vi "Aggregate to Test Suite.vi"(8 "error in (no error)":errorcluster, 11 "Test Finder In":refnum<class "Test Finder.lvclass">) -> (0 "error out":errorcluster, 2 "Test Suite":refnum<class "LUnit Test Suite.lvclass">, 3 "Test Finder Out":refnum<class "Test Finder.lvclass">)   [LabVIEW 2020, in "Test Finder.lvclass"]
uses:
  Test Finder.lvclass
  Test Suite/LUnit Test Suite.lvclass
  Test Finder.lvclass/Test Finder.ctl
  Test Case/LUnit Test Case.lvclass
  Test Case/LUnit Test Case.lvclass/LUnit Test Case.ctl
  Test Suite/LUnit Test Suite.lvclass/LUnit Test Suite.ctl
  Test Case/Public/Accessors/Read Enabled Test Methods.vi
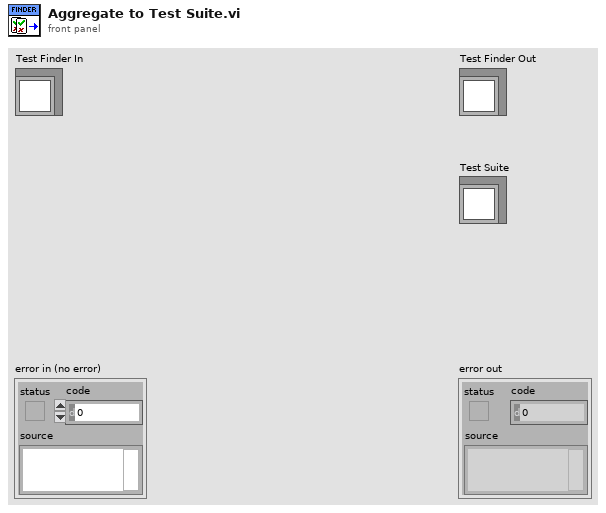
[diagram p1: front panel]
types:
  T1 = map{string, cluster{"Dynamic Methods":map{string, path}, "Static Methods":map{string, path}}}
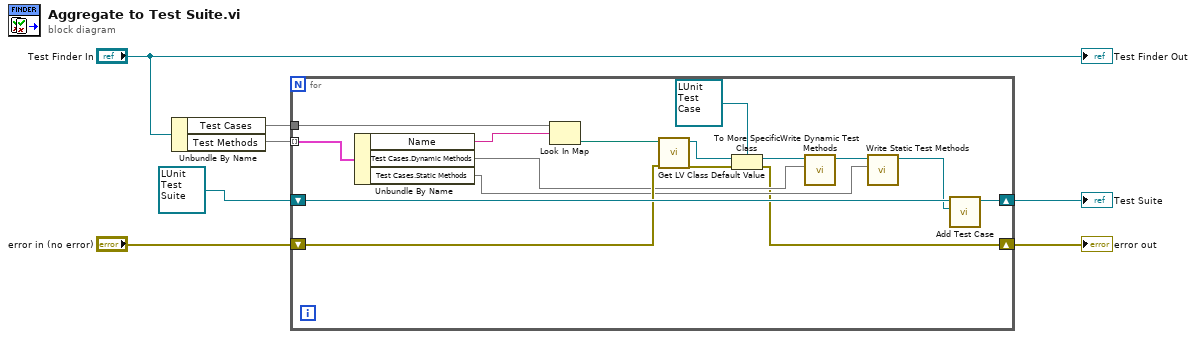
[diagram p0: block diagram]
diagram:
  n1 = Unbundle By Name("Test Finder In") -> ("Test Cases"=w1:map{string, path}, "Test Methods"=w6:T1)
  n2 = for {
    tunnel: w6 -> [w23] mode=indexing
    shift-right: [w22] -> w2
    shift-left: refnum<class "LUnit Test Suite.lvclass"> refnum ("Test Suite.lvclass") -> [w18]
    shift-right: [w8] -> w3
    shift-left: "error in (no error)" -> [w17]
    tunnel: w1 -> [w14]
    n3 = Unbundle By Name(w23) -> ("Name"=w13:string, "Test Cases.Dynamic Methods"=w15:map{string, path}, "Test Cases.Static Methods"=w9:map{string, path})
    n4 = Look In Map(map=w14, key=w13) -> (value=w12:path)  [unwired: 1 in, 1 out]
    n5 = call <vilib>:"Get LV Class Default Value.vi"("error in (no error)"=w17, "class path"=w12) -> ("error out"=w19:errorcluster, "object"=w20:refnum<class>)  [unwired: 8 in]
    n6 = To More Specific Class(target class=refnum<class "LUnit Test Case.lvclass"> refnum ("LUnit Test Case.lvclass"), reference=w20, error in=w19) -> (specific class reference=w16:refnum<class "LUnit Test Case.lvclass">, error out=w8:errorcluster)
    n7 = call "Write Dynamic Test Methods.vi"("Dynamic Test Methods"=w15, "LUnit Test Case In"=w16) -> ("LUnit Test Case Out"=w11:refnum<class "LUnit Test Case.lvclass">)  [unwired: 9 in]
    n8 = call "Write Static Test Methods.vi"("Static Test Methods"=w9, "LUnit Test Case In"=w11) -> ("LUnit Test Case Out"=w10:refnum<class "LUnit Test Case.lvclass">)  [unwired: 9 in]
    n9 = call "Add Test Case.vi"("Test Case to add"=w10, "Test Suite In"=w18) -> ("Test Suite Out"=w22:refnum<class "LUnit Test Suite.lvclass">)  [unwired: 9 in]
  }
  "error out" <- w3
  "Test Suite" <- w2
  "Test Finder Out" <- "Test Finder In"
